vi "FWHM-TEC.vi"(10 "Y values":dbl[](array[numeric]), 11 "WL values":dbl[](array[numeric])) -> (3 "FWHM":dbl)   [LabVIEW 2014]
doc: "Random Laser Project\nAndré Romero - 2020\nandretec@ifsc.usp.br\n\nFWHM - full width at half maximum"
panel:
  out "Right value":dbl
  out "Left value":dbl
  out "Right WL":dbl
  out "min index(es) Right":i32
  out "Left WL":dbl
  out "min index(es) Left":i32
  out "max value / 2":dbl=15982.821433439
  out "WL Center":dbl=600.180869
  out "max index(es)":i32=71
  out "max value":dbl=31965.642866878
  out "XY Graph":cluster{"X Values":dbl[], "Y Values":dbl[]}(graph)={"X Values"=[500.416161, 501.844981, 503.273146, 504.700657, 506.12751, 507.553707, 508.979245, 510.404124, 511.828343, 513.251901, 514.674796, 516.097029, 517.518597, 518.939501, 520.359738, 521.779309, 523.198211, 524.616445, 526.034009, 527.450902, 528.867123, 530.282671, 531.697546, 533.111746, 534.52527, 535.938118, 537.350288, 538.761779, 540.172591, 541.582722, 542.992172, 544.400939, 545.809023, 547.216422, 548.623136, 550.029164, 551.434504, 552.839156, 554.243119, 555.646391, 557.048972, 558.450862, 559.852058, 561.25256, 562.652366, 564.051477, 565.449891, 566.847607, 568.244624, 569.64094, 571.036557, 572.431471, 573.825682, 575.219189, 576.611992, 578.004089, 579.395479, 580.786162, 582.176136, 583.5654, 584.953954, 586.341796, 587.728926, 589.115342, 590.501044, 591.88603, 593.2703, 594.653852, 596.036686, 597.418801, 598.800196, 600.180869, 601.56082, 602.940048, 604.318552, 605.69633, 607.073383, 608.449708, 609.825305, 611.200174, 612.574312, 613.94772, 615.320395, 616.692338, 618.063546, 619.43402, 620.803759, 622.17276, 623.541024, 624.908549, 626.275334, 627.641378, 629.006681, 630.371242, 631.735059, 633.098131, 634.460458, 635.822038, 637.182871, 638.542956, 639.902291, 641.260876, 642.61871, 643.975791, 645.332119, 646.687693, 648.042511, 649.396574, 650.749879, 652.102427, 653.454215, 654.805243, 656.15551, 657.505015, 658.853758, 660.201736, 661.54895, 662.895397, 664.241078, 665.585991, 666.930135, 668.27351, 669.616114, 670.957946, 672.299006, 673.639291, 674.978803, 676.317539, 677.655498, 678.99268, 680.329083, 681.664707, 682.999551, 684.333613, 685.666893, 686.99939, 688.331102, 689.662029, 690.99217, 692.321524, 693.650089, 694.977866, 696.304852, 697.631047, 698.956451], "Y Values"=[28.252866878, -59.127133122, -100.38991112199999, 59.806755878, -10.582689121999996, -20.291578121999997, -25.146022121999998, -20.291578121999997, -20.291578121999997, -5.728244121999998, 28.252866878, 35.534532878, -17.864355122, -13.009911121999997, 59.806755878, -51.845467122, 35.534532878, -0.8738001219999969, -61.554355122, -27.573244122, 47.670644878, 74.370088878, 33.107310878, -0.8738001219999969, -25.146022121999998, 127.768977878, -8.155467122, 11.262310878000003, -30.000467121999996, 52.525088878, -0.8738001219999969, -54.272689122, 18.543977878, 11.262310878000003, 59.806755878, 57.379532878, 86.506199878, 62.233977878, 11.262310878000003, -20.291578121999997, 37.961755878000005, -25.146022121999998, 54.952310878, 37.961755878000005, -37.282133122, 18.543977878, 6.407866878000002, 74.370088878, -0.8738001219999969, 91.360644878, 50.097866878, 96.215088878, 18.543977878, 67.088421878, 154.468421878, 142.332310878, 183.59508887799998, 8.835088878000002, 96.215088878, 144.759532878, 84.078977878, 105.923977878, 127.768977878, 186.02231087799998, 198.15842187799998, 554.960088878, 1656.918977878, 4064.723421878, 9931.319532878, 18875.633421878, 30164.643977878, 31965.642866878, 24448.535644878, 13948.372310878001, 6620.588421877999, 3147.233421878, 1511.285644878, 802.536755878, 453.016755878, 389.90897787800003, 190.87675587799998, 139.905088878, 268.54786687800004, 188.44953287799999, 120.487310878, 152.041199878, -22.718800121999998, 98.642310878, 130.196199878, 156.89564487799998, 76.797310878, 178.74064487799998, 79.224532878, 203.01286687799998, 203.01286687799998, 161.75008887799999, 96.215088878, 125.341755878, 1.5534218780000026, 47.670644878, 62.233977878, -49.418244122, 52.525088878, 13.689532878000001, 8.835088878000002, -17.864355122, 35.534532878, -85.82657812199999, 40.388977878000006, -5.728244121999998, 64.661199878, 62.233977878, 35.534532878, 59.806755878, -34.854911122, 59.806755878, 20.971199878, 11.262310878000003, 127.768977878, -97.96268912199999, -110.09880012199999, -10.582689121999996, 54.952310878, -30.000467121999996, 25.825644878000006, 74.370088878, -27.573244122, 42.816199878, 47.670644878, -32.427689122, 47.670644878, 88.933421878, 18.543977878, 6.407866878000002, 30.680088878, -13.009911121999997, -0.8738001219999969, 86.506199878, 57.379532878, -32.427689122, -5.728244121999998, -68.83602212199999, -20.291578121999997, 11.262310878000003, 52.525088878]}
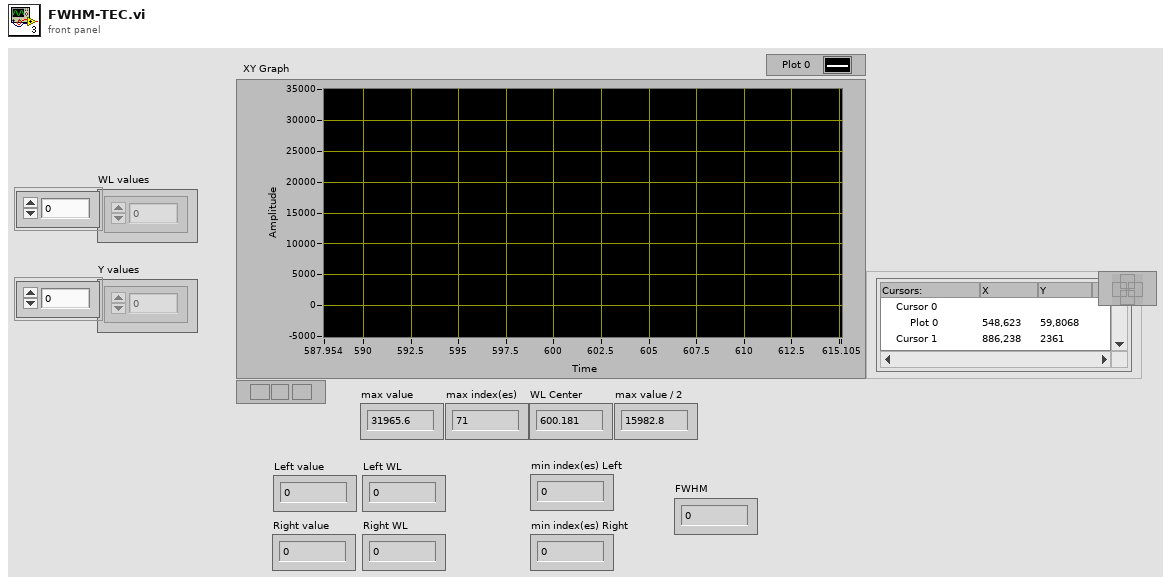
[diagram p1: front panel]
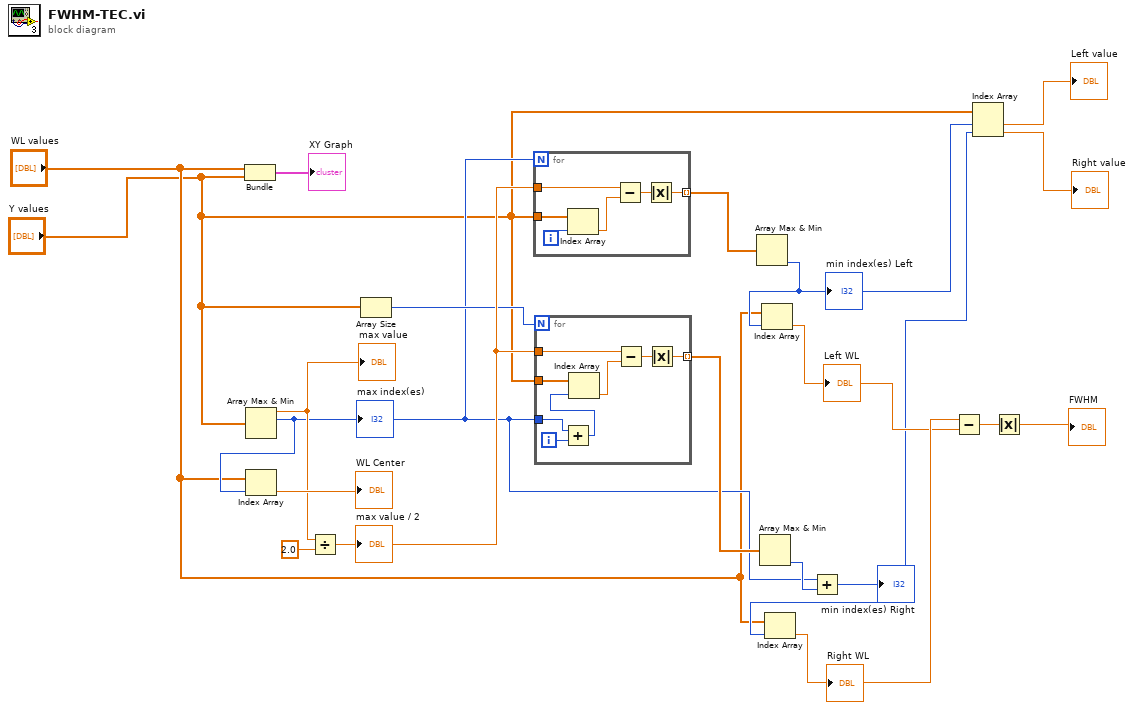
[diagram p0: block diagram]
diagram:
  n1 = Bundle("WL values"="WL values", "Y values"="Y values") -> (→"XY Graph":cluster{"WL values":dbl[], "Y values":dbl[]})  [unwired: 1 in]
  n2 = Array Max & Min(array="Y values") -> (max value=w18:dbl, max index (indices)=w11:i32)  [unwired: 2 out]
  "max value" <- w18
  "max index(es)" <- w11
  n3 = Index Array(array="WL values", index=w11) -> (element=→"WL Center":dbl)
  n4 = Divide(x=w18, y=2.0) -> (x/y=w16:dbl)
  "max value / 2" <- w16
  n5 = Array Size(array="Y values") -> (size(s)=w15:i32)
  n6 = for {
    N: w11 -> [_]
    tunnel: "Y values" -> [w26]
    tunnel: w16 -> [w24]
    tunnel: [w21] -> w14 mode=indexing
    i -> [w25]
    n7 = Index Array(array=w26, index=w25) -> (element=w23:dbl)
    n8 = Subtract(x=w24, y=w23) -> (x-y=w22:dbl)
    n9 = Absolute Value(x=w22) -> (abs(x)=w21:dbl)
  }
  n10 = for {
    N: w15 -> [_]
    tunnel: "Y values" -> [w34]
    tunnel: w16 -> [w33]
    tunnel: [w30] -> w13 mode=indexing
    tunnel: w11 -> [w28]
    i -> [w29]
    n11 = Add(x=w28, y=w29) -> (x+y=w27:i32)
    n12 = Index Array(array=w34, index=w27) -> (element=w32:dbl)
    n13 = Subtract(x=w33, y=w32) -> (x-y=w31:dbl)
    n14 = Absolute Value(x=w31) -> (abs(x)=w30:dbl)
  }
  n15 = Array Max & Min(array=w14) -> (min index (indices)=w6:i32)  [unwired: 3 out]
  "min index(es) Left" <- w6
  n16 = Array Max & Min(array=w13) -> (min index (indices)=w12:i32)  [unwired: 3 out]
  n17 = Index Array(array="WL values", index=w6) -> (element=w8:dbl)
  "Left WL" <- w8
  n18 = Add(x=w11, y=w12) -> (x+y=w5:i32)
  "min index(es) Right" <- w5
  n19 = Index Array(array="WL values", index=w5) -> (element=w9:dbl)
  "Right WL" <- w9
  n20 = Subtract(x=w9, y=w8) -> (x-y=w10:dbl)
  n21 = Index Array(array="Y values", index #1=w6, index #2=w5) -> (element #1=→"Left value":dbl, element #2=→"Right value":dbl)
  n22 = Absolute Value(x=w10) -> (abs(x)=→"FWHM":dbl)
